vi "SimpleSetReadExample.vi"() -> ()   [LabVIEW 2023]
panel:
  out "Waveform Chart":T1(graph)
  in  "Stop":bool
  in  "Temperature (°C) 2":dbl min=0.0 max=450.0 step=1.0
  out "Temperature (°C)":dbl min=0.0 max=450.0 step=1.0
  in  "VISA resource name":refnum<visa-resource-name>
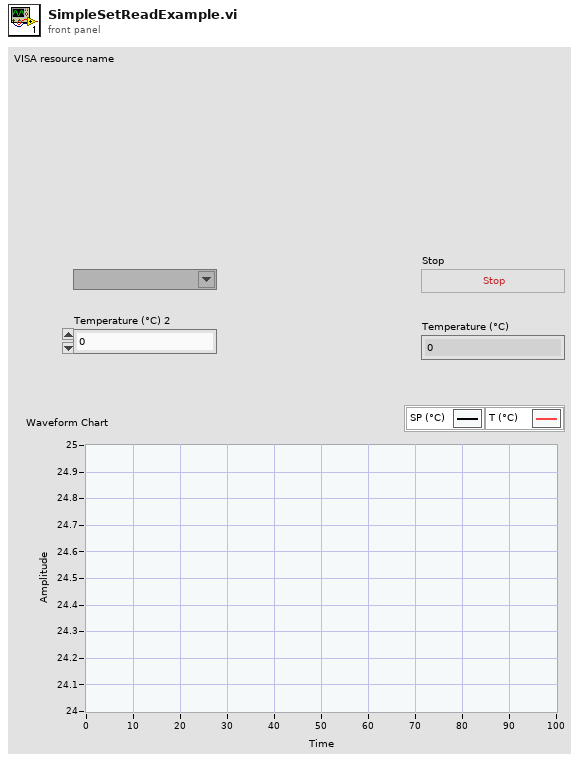
[diagram p1: front panel]
types:
  T1 = cluster{"Temperature (°C)":dbl, "Temperature (°C) 2":dbl}
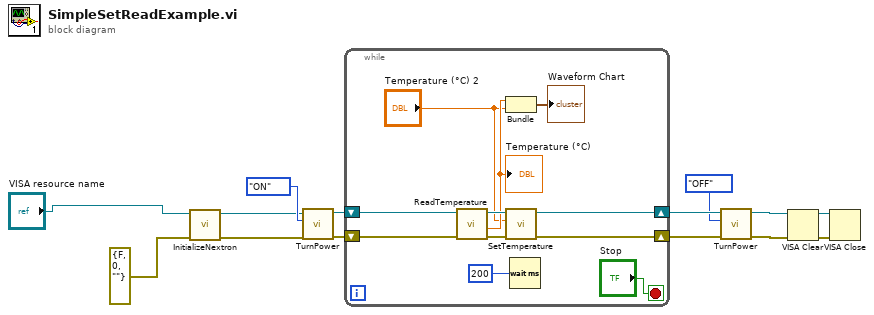
[diagram p0: block diagram]
diagram:
  n1 = call "InitializeNextron.vi"("error in (no error)"=errorcluster {"status"=FALSE, "code"=0, "source"=""}, "VISA Refnum in"="VISA resource name") -> ("error in (no error) 2"=w1:errorcluster, "VISA Refnum Out"=w2:refnum<visa-resource-name>)  [unwired: 7 in, 1 out]
  n2 = call "TurnPower.vi"("error in (no error)"=w1, "Power ON/OFF"=enum16{"ON", "OFF"}."ON", "VISA Refnum in"=w2) -> ("error in (no error) 2"=w12:errorcluster, "VISA Refnum Out"=w13:refnum<visa-resource-name>)  [unwired: 7 in]
  n3 = while {
    shift-right: [w20] -> w6
    shift-left: w13 -> [w25]
    shift-right: [w21] -> w9
    shift-left: w12 -> [w24]
    stop <- "Stop" stop-if-true
    n4 = call "ReadTemperature.vi"("error in (no error)"=w24, "VISA Refnum in"=w25) -> ("error in (no error) 2"=w22:errorcluster, "Temperature (°C)"=w18:dbl, "VISA Refnum Out"=w23:refnum<visa-resource-name>)  [unwired: 6 in, 1 out]
    "Temperature (°C)" <- w18
    n5 = Bundle("Temperature (°C)"=w18, "Temperature (°C) 2"="Temperature (°C) 2") -> (→"Waveform Chart":T1)  [unwired: 1 in]
    n6 = call "SetTemperature.vi"("error in (no error)"=w22, "Temperature (°C)"="Temperature (°C) 2", "VISA Refnum in"=w23) -> ("error in (no error) 2"=w21:errorcluster, "VISA Refnum Out"=w20:refnum<visa-resource-name>)  [unwired: 7 in]
    n7 = Wait (ms)(milliseconds to wait=u32 200) -> ()  [unwired: 1 out]
  }
  n8 = call "TurnPower.vi"("error in (no error)"=w9, "Power ON/OFF"=enum16{"ON", "OFF"}."OFF", "VISA Refnum in"=w6) -> ("error in (no error) 2"=w8:errorcluster, "VISA Refnum Out"=w7:refnum<visa-resource-name>)  [unwired: 7 in]
  n9 = VISA Clear(VISA resource name=w7, error in (no error)=w8) -> (VISA resource name out=w11:refnum<visa-resource-name>, error out=w10:errorcluster)
  n10 = VISA Close(VISA resource name=w11, error in (no error)=w10) -> ()  [unwired: 1 out]
